vi "Pre-Process.vi"(11 "Asteroid in":refnum<class "Asteroid.lvclass">) -> (3 "Asteroid out":refnum<class "Asteroid.lvclass">)   [LabVIEW 2021, in "Asteroid.lvclass"]
uses:
  Asteroid.lvclass
  C:/dev/LabVIEW/LabMelee/Source/Application Specific/Element/Element.lvclass
  Asteroid.lvclass/Asteroid.ctl
  <vilib>/numeric/Random Number (Range) DBL.vi
  Re-use Libraries/Vector 2D/Initialise.vi
  Element/Element.lvclass
  Re-use Libraries/Vector 2D/Vector 2D.lvclass
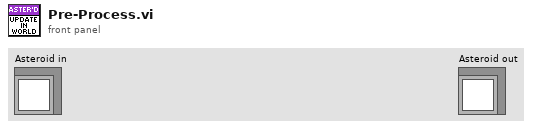
[diagram p1: front panel]
types:
  T1 = typedef "Constants.ctl" = cluster{"Colours":cluster{"OK":u32, "Warning":u32, "Error":u32, "Red":u32, "Green":u32, "Blue":u32, "Yellow":u32}, "System":cluster{"Target Frames Second":dbl, "Windows Size":refnum<class "Vector 2D.lvclass">, "World Size":refnum<class "Vector 2D.lvclass">, "Battle Area Size":refnum<class "Vector 2D.lvclass">, "Sidebar Width":sgl, "SC2 Frame Rate [Seconds/Frame]":sgl, "Sidebar Player 2 Y Offset":sgl}, "Game":cluster{"Maximum Asteroids":i32, "Max Energy":i32, "Max Crew":i32, "Maximum Stars":i32}}
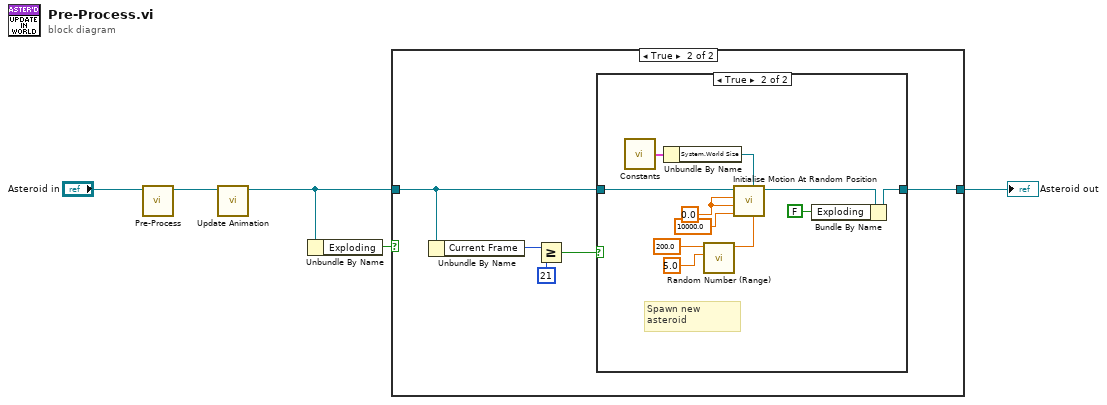
[diagram p0: block diagram]
diagram:
  n1 = call-parent "Pre-Process.vi"("Element in"="Asteroid in") -> ("Element out"=w4:refnum<class "Asteroid.lvclass">)  [unwired: 10 in]
  n2 = call "Update Animation.vi"("Asteroid in"=w4) -> ("Asteroid out"=w2:refnum<class "Asteroid.lvclass">)  [unwired: 10 in]
  n3 = Unbundle By Name(w2) -> ("Exploding"=w3:bool)
  n4 = case shown="True" w3 {
    tunnel: [w6 w8] -> w1
    tunnel: w2 -> [w6 w11]
    frame False {
    }
    frame True {
      n5 = Unbundle By Name(w11) -> ("Current Frame"=w7:i32)
      n6 = Greater Or Equal?(x=w7, y=21) -> (x >= y?=w9:bool)
      n7 = case shown="True" w9 {
        tunnel: [w12 w19] -> w8
        tunnel: w11 -> [w12 w23]
        frame False {
        }
        frame True {
          w22 = sgl 0.0 ("Turn Rate [deg/s]")
          # "Spawn new asteroid"
          n8 = call "Constants.vi"() -> ("Constants"=w17:T1)
          n9 = Unbundle By Name(w17) -> ("System.World Size"=w21:refnum<class "Vector 2D.lvclass">)
          n10 = call-poly <vilib>:"Random Number (Range).vi"("lower bound (0)"=sgl 5.0 ("Initial Heading [deg]"), "upper bound (100)"=sgl 200.0 ("Initial Heading [deg]")) -> ("number"=w14:dbl)  [unwired: 9 in]
          n11 = call "Initialise Motion At Random Position.vi"("Initial Velocity [m/s]"=w14, "Field Size"=w21, "Maximum Velocity [m/s]"=sgl 10000.0, "Acceleration [m/s/s]"=w22, "Turn Rate [deg/s]"=w22, "Element in"=w23) -> ("Element out"=w20:refnum<class "Asteroid.lvclass">)  [unwired: 5 in]
          n12 = Bundle By Name(cluster=w20, "Exploding"=FALSE) -> (w19:refnum<class "Asteroid.lvclass">)
        }
      }
    }
  }
  "Asteroid out" <- w1
